vi "SP_REJECTION_Count_DayWise12.vi"(8 "Shift":string(combo), 9 "Select Station":string(combo), 10 "To Date":timestamp format="%<%Y-%m-%d>T", 11 "From Date":timestamp format="%<%Y-%m-%d>T") -> (3 "Table":string[][](table))   [LabVIEW 2017]
uses:
  <vilib>/Math Plots/3D Math Plots/3D Pie/3D Pie XCtrl/3D Pie.xctl
  <vilib>/addons/database/Connection.llb/DB Tools Open Connec (Path).vi
  <vilib>/Math Plots/3D Math Plots/3D Pie/3D Pie Datatype/Public/Plot Helper (Vector).vi
  <vilib>/addons/database/NI_Database_API.lvlib
  <vilib>/Math Plots/3D Math Plots/3D Pie/3D Pie Datatype/3D Pie Datatype.lvclass
panel:
  in  "Cancel Button - Archive":bool
  in  "Get Rport 2":bool
  in  "Download 2":bool
  out "error out":errorcluster
  out "sum":i32[](array[numeric])
  out "Table 3":string[][](array[string])
  out "heading 1":string="Gap Leader"
  out "heading2":string="Logistics"
  out "heading 3":string="Maintenance"
  out "heading 4":string="Qaulity"
  out "heading 5":string="Production"
  out "heading 6":string="Total"
  in  "error in (no error)":errorcluster
  in  "Tab Control":enum32{"Data", "Graph"}(tab)
  out "Table ALL":string[][](table)
  out "250T-3 Total":i32
  out "250T-2 Total":i32
  out "250T-1 Total":i32
  out "400T-1 Total":i32
  out "150T-1 Total":i32
  out "400T-2 Total":i32
  out "All Total":i32
  out "3D Pie":refnum<class "3D Plot Datatype.lvclass">[](xcontrol)
  in  "Select Stakeholder":string(combo)
  # "Date"
  # "All Station"
  # "Station 1"
  # "Station 2"
  # "Station 3"
  # "Station 4"
  # "Station 5"
  # "Station 6"
  # "Rejection Count Report"
  # "Total"
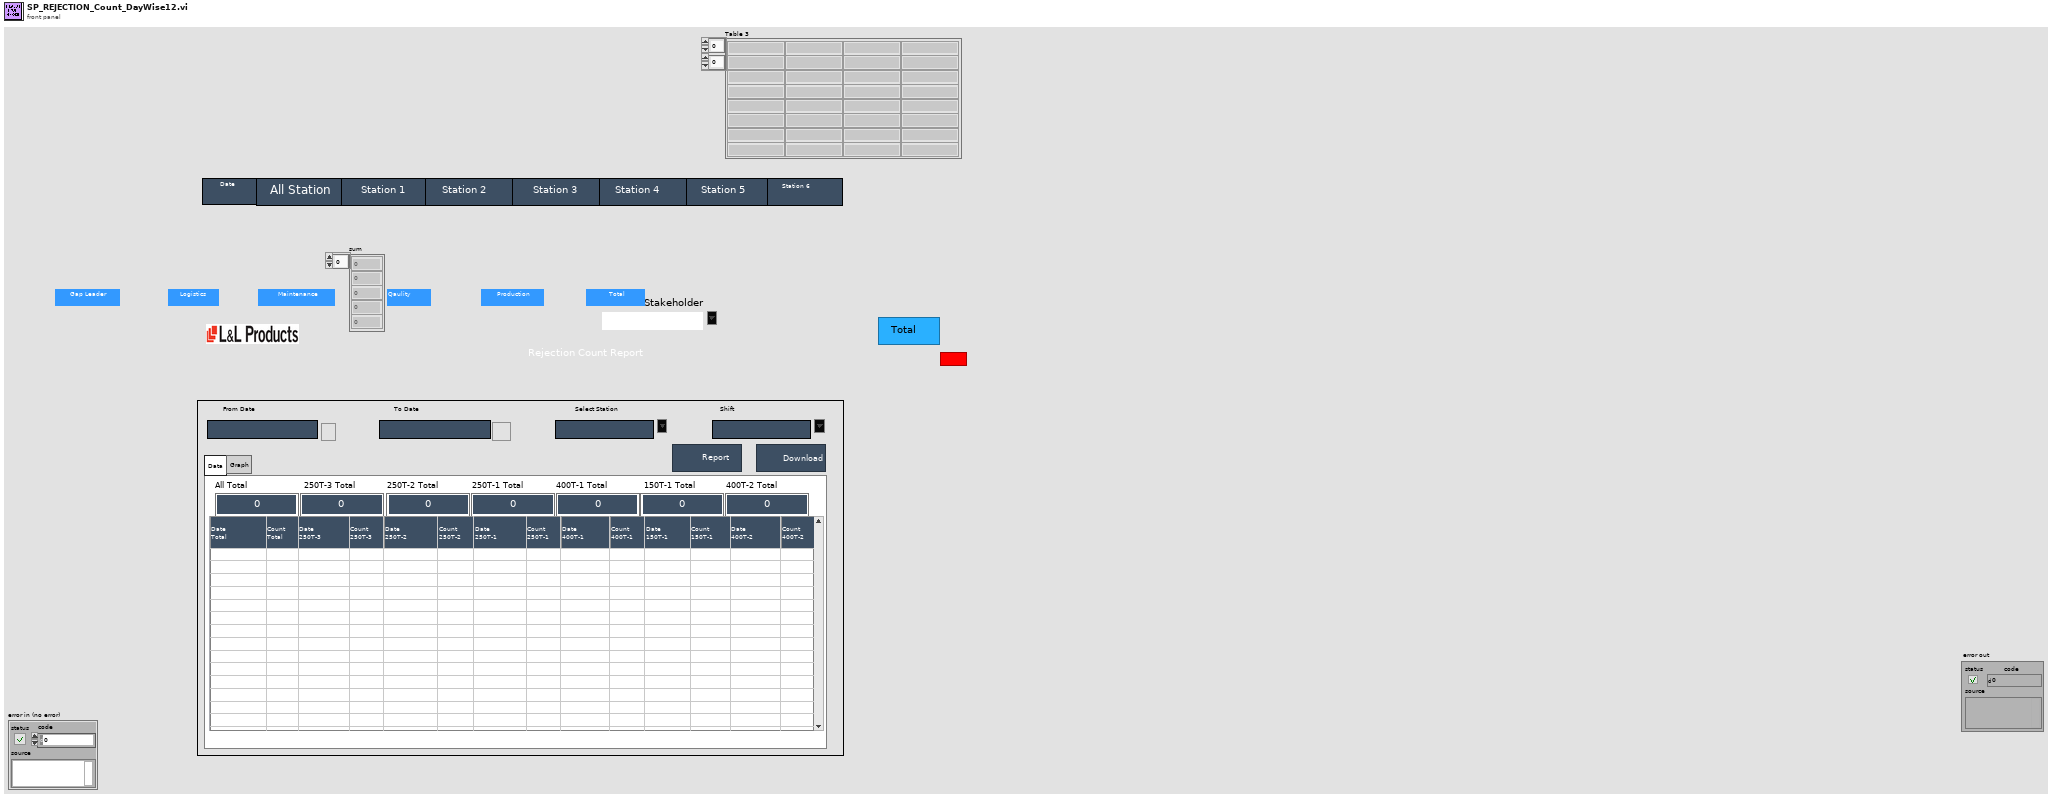
[diagram p1: front panel]
types:
  T1 = typedef "NI_Database_API.lvlib/Conn ObjectReference.ctl" = refnum<k1>
  T2 = enum32{"invalid app kind", "Development System", "Run Time System", "Student Edition", "Embedded LabVIEW", "Evaluation", "Custom"}
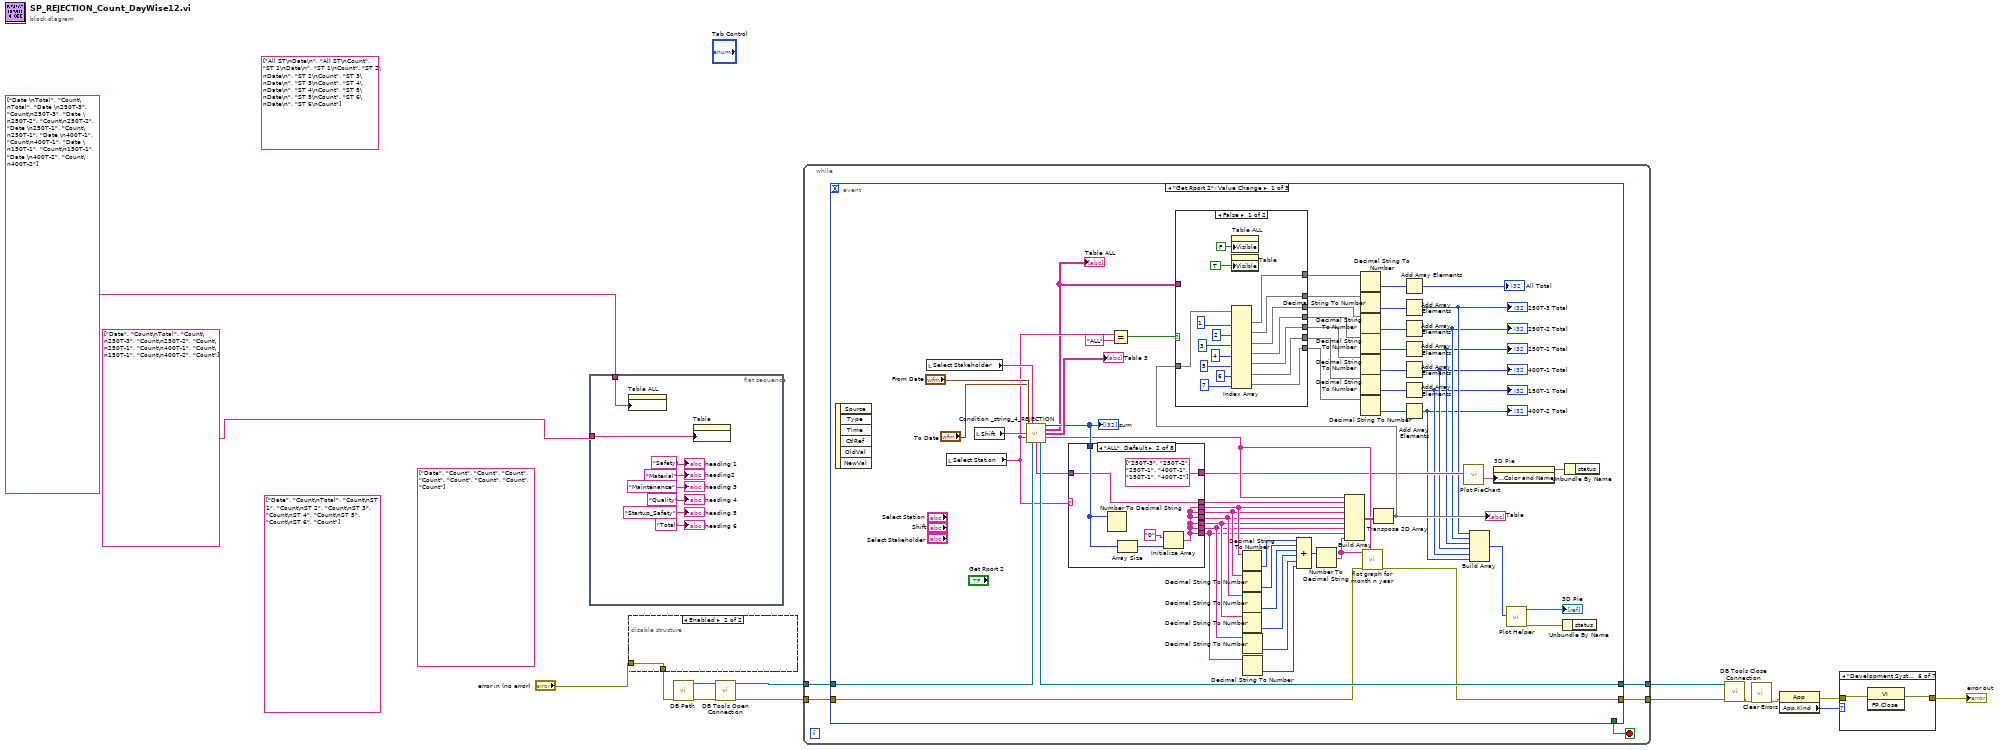
[diagram p0: block diagram]
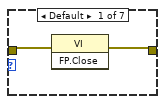
[diagram p2: hidden frame]
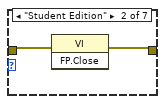
[diagram p3: hidden frame]
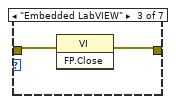
[diagram p4: hidden frame]
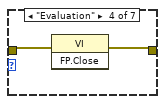
[diagram p5: hidden frame]
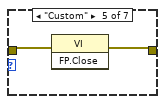
[diagram p6: hidden frame]
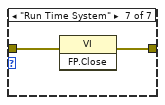
[diagram p7: hidden frame]
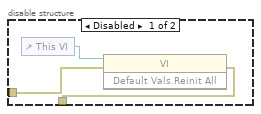
[diagram p8: hidden frame]
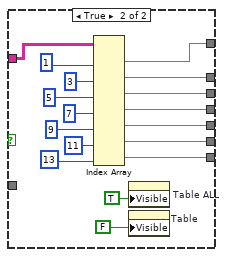
[diagram p9: hidden frame]
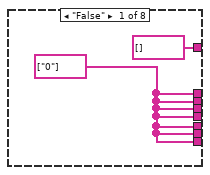
[diagram p10: hidden frame]
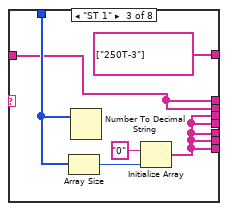
[diagram p11: hidden frame]
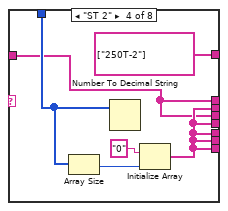
[diagram p12: hidden frame]
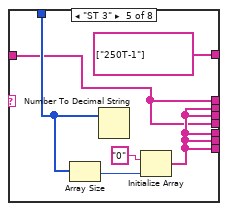
[diagram p13: hidden frame]
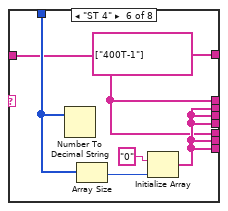
[diagram p14: hidden frame]
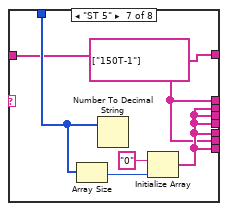
[diagram p15: hidden frame]
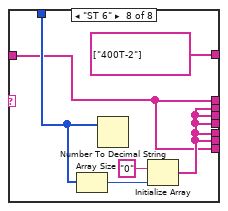
[diagram p16: hidden frame]
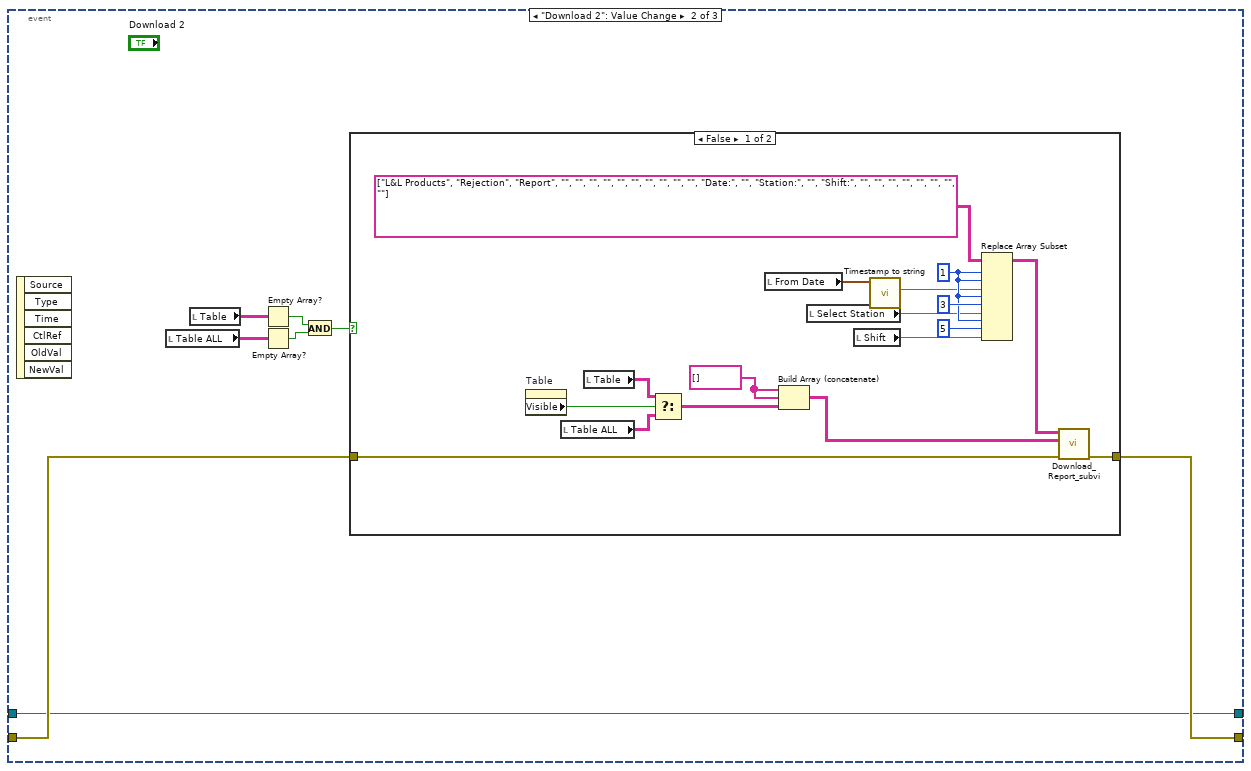
[diagram p17: hidden frame]
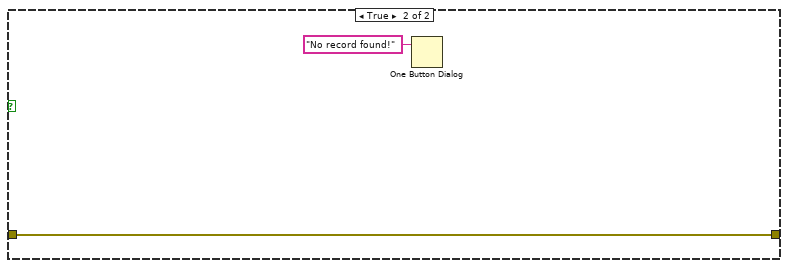
[diagram p18: hidden frame]
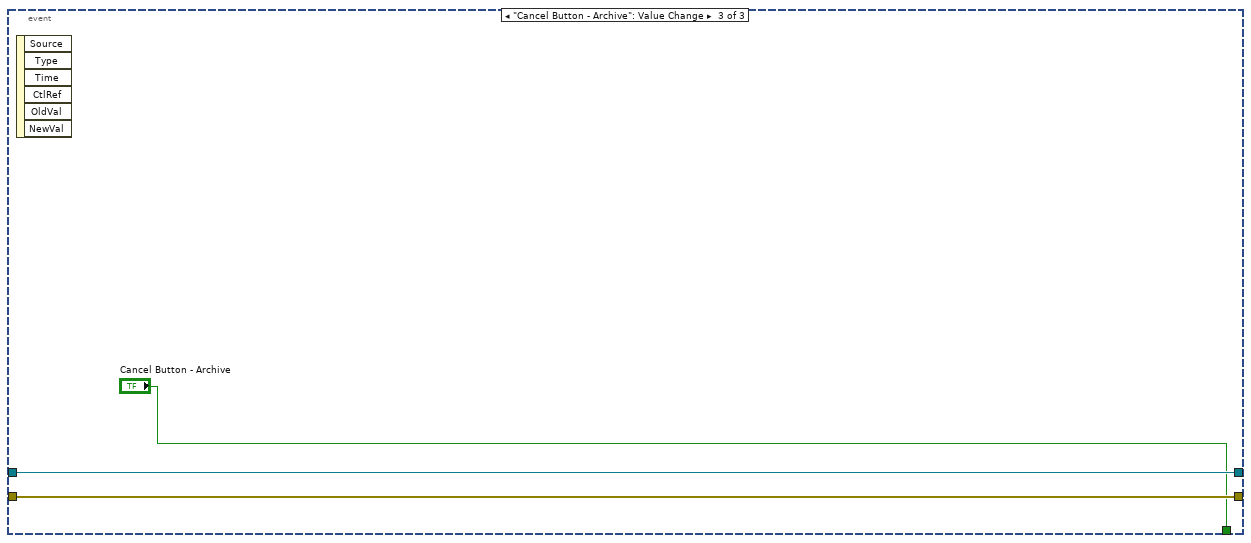
[diagram p19: hidden frame]
diagram:
  (unwired) string[] ["Date", "Count\nTotal", "Count\nST 1", "Count\nST 2", "Count\nST 3", "Count\nST 4", "Count\nST 5", "Count\nST 6", "Count"] ("Column Header Strings[]")
  (unwired) string[] ["All ST\nDate\n", "All ST\nCount", "ST 1\nDate\n", "ST 1\nCount", "ST 2\nDate\n", "ST 2\nCount", "ST 3\nDate\n", "ST 3\nCount", "ST 4\nDate\n", "ST 4\nCount", "ST 5\nDate\n", "ST 5\nCount", "ST 6\nDate\n", "ST 6\nCount"] ("Column Header Strings[]")
  (unwired) string[] ["Date", "Count", "Count", "Count", "Count", "Count", "Count", "Count", "Count"] ("Column Header Strings[]")
  n1 = flat-sequence {
    tunnel: string[] ["Date", "Count\nTotal", "Count\n250T-3", "Count\n250T-2", "Count\n250T-1", "Count\n400T-1", "Count\n150T-1", "Count\n400T-2", "Count"] ("Column Header Strings[]") -> [w17]
    tunnel: string[] ["Date \nTotal", "Count\nTotal", "Date \n250T-3", "Count\n250T-3", "Date \n250T-2", "Count\n250T-2", "Date \n250T-1", "Count\n250T-1", "Date \n400T-1", "Count\n400T-1", "Date \n150T-1", "Count\n150T-1", "Date \n400T-2", "Count\n400T-2"] ("Column Header Strings[]") -> [w16]
    frame #0 {
      n2 = property on="Table ALL" class="Tbl (strict)"("Column Headers[]"=w16) -> ()  [unwired: 2 in, 2 out]
      n3 = property on="Table" class="Tbl (strict)"("Column Headers[]"=w17) -> ()  [unwired: 2 in, 2 out]
      "heading 1" <- "Safety" ("heading 1")
      "heading2" <- "Material" ("heading2")
      "heading 3" <- "Maintenance" ("heading 3")
      "heading 4" <- "Quality" ("heading 4")
      "heading 5" <- "Startup_Safety" ("heading 5")
      "heading 6" <- "Total" ("heading 6")
    }
  }
  n4 = disable-structure shown="Enabled" {
    disable-tunnel: "error in (no error)" -> [w25 w27]
    disable-tunnel: [w24 w27] -> w12
    frame Disabled {
      n5 = control-ref of="This VI"() -> (w26:refnum<vi>)
      n6 = invoke class="VI" method="Default Vals.Reinit All"(reference=w26, error in=w25) -> (error out=w24:errorcluster)  [unwired: 1 in, 2 out]
    }
    frame Enabled {
    }
  }
  n7 = call "DB Path.vi"("error in"=w12) -> ("error out"=w15:errorcluster, "DB Path"=w14:path)  [unwired: 9 in]
  n8 = call-poly <vilib>:"DB Tools Open Connection.vi"("error in (no error)"=w15, "connection information"=w14) -> ("error out"=w11:errorcluster, "connection reference"=w10:T1)  [unwired: 6 in]
  n9 = while {
    tunnel: w11 -> [w32]
    tunnel: w10 -> [w31]
    tunnel: [w30] -> w4
    tunnel: [w29] -> w3
    stop <- w28 stop-if-true
    n10 = event shown="[0] \"Get Rport 2\": Value Change" {
      selector: _ -> [_ _ _]
      dyn-events: _ -> [_ _ _]
      timeout: _ -> [_ _ _]
      tunnel: w32 -> [w81 w178 w200]
      tunnel: w31 -> [w83 w176 w199]
      tunnel: [w80 w177 w200] -> w30
      tunnel: [w82 w176 w199] -> w29
      tunnel: [_ _ "Cancel Button - Archive"] -> w28
      event "Get Rport 2": Value Change {
        n11 = event-data() -> ()  [unwired: 1 in, 6 out]
        n12 = local read "Select Stakeholder"() -> (w85:string)
        n13 = local read "Select Station"() -> (w78:string)
        n14 = local read "Shift"() -> (w90:string)
        n15 = call "Condition _string_4_REJECTION.vi"("From Date"="From Date", "Select Stakeholder"=w85, "To Date"="To Date", "Shift"=w90, "Select Station"=w78, "Refnum out 2"=w83) -> ("sum"=w88:i32[], "all station"=w63:string[][], "Table"=→"Table 3":string[][], "Elements Found out"=w56:string[], "PROD_COUNT TEST"=w79:string[], "Refnum out"=w82:T1)  [unwired: 2 in, 2 out]
        "sum" <- w88
        "Table ALL" <- w63
        n16 = case shown="\"ALL\", Default" w78 {
          tunnel: w88 -> [_ w134 w138 w144 w150 w156 w162 w168]
          tunnel: [w128 w130 w136 w142 w148 w154 w160 w166] -> w86
          tunnel: [w128 w131 w136 w143 w149 w155 w161 w167] -> w51
          tunnel: [w128 w131 w137 w142 w149 w155 w161 w167] -> w50
          tunnel: [w128 w131 w137 w143 w148 w155 w161 w167] -> w49
          tunnel: [w128 w131 w137 w143 w149 w154 w161 w167] -> w48
          tunnel: [w128 w131 w137 w143 w149 w155 w160 w167] -> w47
          tunnel: [w128 w131 w137 w143 w149 w155 w161 w166] -> w46
          tunnel: w79 -> [_ w130 w136 w142 w148 w154 w160 w166]
          tunnel: [string[] [] string[] ["250T-3", "250T-2", "250T-1", "400T-1", "150T-1", "400T-2"] string[] ["250T-3"] string[] ["250T-2"] string[] ["250T-1"] string[] ["400T-1"] string[] ["150T-1"] string[] ["400T-2"]] -> w52
          frame "False" {
            w128 = string[] ["0"]
          }
          frame "ALL", Default {
            n17 = Number To Decimal String(number=w134) -> ()  [unwired: 1 in, 1 out]
            n18 = Array Size(array=w134) -> (size(s)=w133:i32)
            n19 = Initialize Array("0", w133) -> (w131:string[])
          }
          frame "ST 1" {
            n20 = Array Size(array=w138) -> (size(s)=w140:i32)
            n21 = Number To Decimal String(number=w138) -> ()  [unwired: 1 in, 1 out]
            n22 = Initialize Array("0", w140) -> (w137:string[])
          }
          frame "ST 2" {
            n23 = Array Size(array=w144) -> (size(s)=w146:i32)
            n24 = Number To Decimal String(number=w144) -> ()  [unwired: 1 in, 1 out]
            n25 = Initialize Array("0", w146) -> (w143:string[])
          }
          frame "ST 3" {
            n26 = Array Size(array=w150) -> (size(s)=w152:i32)
            n27 = Number To Decimal String(number=w150) -> ()  [unwired: 1 in, 1 out]
            n28 = Initialize Array("0", w152) -> (w149:string[])
          }
          frame "ST 4" {
            n29 = Number To Decimal String(number=w156) -> ()  [unwired: 1 in, 1 out]
            n30 = Array Size(array=w156) -> (size(s)=w158:i32)
            n31 = Initialize Array("0", w158) -> (w155:string[])
          }
          frame "ST 5" {
            n32 = Array Size(array=w162) -> (size(s)=w164:i32)
            n33 = Number To Decimal String(number=w162) -> ()  [unwired: 1 in, 1 out]
            n34 = Initialize Array("0", w164) -> (w161:string[])
          }
          frame "ST 6" {
            n35 = Array Size(array=w168) -> (size(s)=w170:i32)
            n36 = Number To Decimal String(number=w168) -> ()  [unwired: 1 in, 1 out]
            n37 = Initialize Array("0", w170) -> (w167:string[])
          }
        }
        n38 = Equal?(x=w78, y="ALL") -> (x = y?=w76:bool)
        n39 = Decimal String To Number(string=w51) -> (number=w45:i32[])  [unwired: 2 in, 1 out]
        n40 = Decimal String To Number(string=w50) -> (number=w44:i32[])  [unwired: 2 in, 1 out]
        n41 = Decimal String To Number(string=w49) -> (number=w43:i32[])  [unwired: 2 in, 1 out]
        n42 = Decimal String To Number(string=w48) -> (number=w42:i32[])  [unwired: 2 in, 1 out]
        n43 = Decimal String To Number(string=w47) -> (number=w41:i32[])  [unwired: 2 in, 1 out]
        n44 = Decimal String To Number(string=w46) -> (number=w40:i32[])  [unwired: 2 in, 1 out]
        n45 = Compound Arithmetic op=ADD(w45, w44, w43, w42, w41, w40) -> (w53:i32[])
        n46 = Number To Decimal String(number=w53) -> (decimal integer string=w84:string[])  [unwired: 1 in]
        n47 = Build Array(w56, w86, w51, w50, w49, w48, w47, w46, w84) -> (w87:string[][])
        n48 = call "flot graph for month n year.vi"("BD Date"=w56, "error in (no error)"=w81, "Count total"=w84) -> ("error out"=w80:errorcluster)  [unwired: 7 in, 1 out]
        n49 = Transpose 2D Array(2D array=w87) -> (transposed array=w59:string[][])
        "Table" <- w59
        n50 = case shown="False" w76 {
          tunnel: w63 -> [_ w120]
          tunnel: [w98 w119] -> w69
          tunnel: [w97 w118] -> w68
          tunnel: [w96 w117] -> w67
          tunnel: [w95 w116] -> w66
          tunnel: [w94 w115] -> w65
          tunnel: [w93 w114] -> w64
          tunnel: [w99 w110] -> w62
          tunnel: w59 -> [w100 _]
          frame False {
            n51 = Index Array(array=w100, index (col) #1=1 ("disabled index (col)"), index (col) #2=2 ("disabled index (col)"), index (col) #3=3 ("disabled index (col)"), index (col) #4=4 ("disabled index (col)"), index (col) #5=5 ("disabled index (col)"), index (col) #6=6 ("disabled index (col)"), index (col) #7=7 ("disabled index (col)")) -> (element #1=w99:string[], element #2=w98:string[], element #3=w97:string[], element #4=w96:string[], element #5=w95:string[], element #6=w94:string[], element #7=w93:string[])  [unwired: 7 in]
            n52 = property on="Table ALL" class="Tbl (strict)"("Visible"=FALSE) -> ()  [unwired: 2 in, 2 out]
            n53 = property on="Table" class="Tbl (strict)"("Visible"=TRUE) -> ()  [unwired: 2 in, 2 out]
          }
          frame True {
            n54 = Index Array(array=w120, index (col) #1=1 ("disabled index (col)"), index (col) #2=3 ("disabled index (col)"), index (col) #3=5 ("disabled index (col)"), index (col) #4=7 ("disabled index (col)"), index (col) #5=9 ("disabled index (col)"), index (col) #6=11 ("disabled index (col)"), index (col) #7=13 ("disabled index (col)")) -> (element #1=w110:string[], element #2=w119:string[], element #3=w118:string[], element #4=w117:string[], element #5=w116:string[], element #6=w115:string[], element #7=w114:string[])  [unwired: 7 in]
            n55 = property on="Table ALL" class="Tbl (strict)"("Visible"=TRUE) -> ()  [unwired: 2 in, 2 out]
            n56 = property on="Table" class="Tbl (strict)"("Visible"=FALSE) -> ()  [unwired: 2 in, 2 out]
          }
        }
        n57 = Decimal String To Number(string=w62) -> (number=w61:i32[])  [unwired: 2 in, 1 out]
        n58 = Decimal String To Number(string=w69) -> (number=w70:i32[])  [unwired: 2 in, 1 out]
        n59 = Decimal String To Number(string=w68) -> (number=w71:i32[])  [unwired: 2 in, 1 out]
        n60 = Decimal String To Number(string=w67) -> (number=w72:i32[])  [unwired: 2 in, 1 out]
        n61 = Decimal String To Number(string=w66) -> (number=w73:i32[])  [unwired: 2 in, 1 out]
        n62 = Decimal String To Number(string=w65) -> (number=w74:i32[])  [unwired: 2 in, 1 out]
        n63 = Decimal String To Number(string=w64) -> (number=w75:i32[])  [unwired: 2 in, 1 out]
        n64 = Add Array Elements(numeric array=w61) -> (sum=→"All Total":i32)
        n65 = Add Array Elements(numeric array=w70) -> (sum=w38:i32)
        "250T-3 Total" <- w38
        n66 = Add Array Elements(numeric array=w71) -> (sum=w37:i32)
        "250T-2 Total" <- w37
        n67 = Add Array Elements(numeric array=w72) -> (sum=w36:i32)
        "250T-1 Total" <- w36
        n68 = Add Array Elements(numeric array=w73) -> (sum=w35:i32)
        "400T-1 Total" <- w35
        n69 = Add Array Elements(numeric array=w74) -> (sum=w34:i32)
        "150T-1 Total" <- w34
        n70 = Add Array Elements(numeric array=w75) -> (sum=w33:i32)
        "400T-2 Total" <- w33
        n71 = call "Plot PieChart.vi"("Label"=w52) -> ("Labelling"=w57:cluster{dbl, "String":string}[])  [unwired: 10 in]
        n72 = Build Array(w38, w37, w36, w35, w34, w33) -> (w39:i32[])
        n73 = property on="3D Pie" class="3D Pie (strict)"("Plot Specific:Color and Name"=w57) -> (error out=w58:errorcluster)  [unwired: 2 in, 1 out]
        n74 = call-poly <vilib>:"Plot Helper.vi"("x vector"=w39) -> ("error out"=w55:errorcluster, "3D Plot lvclass Array out"=→"3D Pie":refnum<class "3D Plot Datatype.lvclass">[])  [unwired: 2 in, 7 out]
        n75 = Unbundle By Name(w55) -> ()  [unwired: 1 out]
        n76 = Unbundle By Name(w58) -> ()  [unwired: 1 out]
      }
      event "Download 2": Value Change {
        n77 = event-data() -> ()  [unwired: 1 in, 6 out]
        n78 = local read "Table ALL"() -> (w171:string[][])
        n79 = local read "Table"() -> (w173:string[][])
        n80 = Empty Array?(array=w173) -> (empty?=w174:bool)
        n81 = Empty Array?(array=w171) -> (empty?=w172:bool)
        n82 = And(x=w174, y=w172) -> (x .and. y?=w175:bool)
        n83 = case shown="False" w175 {
          tunnel: w178 -> [w195 w197]
          tunnel: [w194 w197] -> w177
          frame False {
            w183 = string[] [] ("element")
            w192 = 1 ("index (row)")
            n84 = property on="Table" class="Tbl (strict)"() -> ("Visible"=w182:bool)  [unwired: 2 in, 2 out]
            n85 = local read "Table ALL"() -> (w179:string[][])
            n86 = local read "Table"() -> (w181:string[][])
            n87 = Select(t=w181, s=w182, f=w179) -> (s? t:f=w180:string[][])
            n88 = local read "From Date"() -> (w189:timestamp)
            n89 = Build Array (concatenate)(w183, w183, w180) -> (w184:string[][])
            n90 = local read "Select Station"() -> (w186:string)
            n91 = local read "Shift"() -> (w187:string)
            n92 = call "Timestamp to string.vi"("time stamp"=w189) -> ("Date"=w188:string)  [unwired: 8 in, 2 out]
            n93 = Replace Array Subset(array=string[][] [["L&L Products", "Rejection", "Report", "", "", "", "", "", "", "", "", "", ""], ["Date:", "", "Station:", "", "Shift:", "", "", "", "", "", "", "", ""]] ("Column Header Strings[]"), new element #1=w188, index (row) #1=w192, index (col) #1=w192, new element #2=w186, index (row) #2=w192, index (col) #2=3 ("disabled index (col)"), new element #3=w187, index (row) #3=w192, index (col) #3=5 ("disabled index (col)")) -> (w185:string[][])
            n94 = call "Download_Report_subvi.vi"("error in (no error)"=w195, "Value"=w184, "Column Header Strings[]"=w185) -> ("error out"=w194:errorcluster)  [unwired: 8 in]
          }
          frame True {
            n95 = One Button Dialog(message="No record found!") -> ()  [unwired: 1 in, 1 out]
          }
        }
      }
      event "Cancel Button - Archive": Value Change {
        n96 = event-data() -> ()  [unwired: 1 in, 6 out]
      }
    }
  }
  n97 = call <vilib>:"DB Tools Close Connection.vi"("error in (no error)"=w4, "connection reference"=w3) -> ("error out"=w6:errorcluster)  [unwired: 5 in]
  n98 = call <vilib>:"Clear Errors.vi"("error in (no error)"=w6) -> ("error out"=w5:errorcluster)  [unwired: 5 in, 1 out]
  n99 = property class="App"(error in=w5) -> (error out=w8:errorcluster, "App.Kind"=w9:T2)  [unwired: 1 in, 1 out]
  n100 = case shown="\"Development System\"" w9 {
    tunnel: w8 -> [w202 w204 w206 w208 w210 w212 w214]
    tunnel: [w201 w203 w205 w207 w209 w211 w213] -> w7
    frame Default {
      n101 = invoke class="VI" method="FP.Close"(error in=w202) -> (error out=w201:errorcluster)  [unwired: 2 in, 2 out]
    }
    frame "Student Edition" {
      n102 = invoke class="VI" method="FP.Close"(error in=w204) -> (error out=w203:errorcluster)  [unwired: 2 in, 2 out]
    }
    frame "Embedded LabVIEW" {
      n103 = invoke class="VI" method="FP.Close"(error in=w206) -> (error out=w205:errorcluster)  [unwired: 2 in, 2 out]
    }
    frame "Evaluation" {
      n104 = invoke class="VI" method="FP.Close"(error in=w208) -> (error out=w207:errorcluster)  [unwired: 2 in, 2 out]
    }
    frame "Custom" {
      n105 = invoke class="VI" method="FP.Close"(error in=w210) -> (error out=w209:errorcluster)  [unwired: 2 in, 2 out]
    }
    frame "Development System" {
      n106 = invoke class="VI" method="FP.Close"(error in=w212) -> (error out=w211:errorcluster)  [unwired: 2 in, 2 out]
    }
    frame "Run Time System" {
      n107 = invoke class="VI" method="FP.Close"(error in=w214) -> (error out=w213:errorcluster)  [unwired: 2 in, 2 out]
    }
  }
  "error out" <- w7
